vi "openCamera.vi"(0 "error in":errorcluster, 2 "Camera Settings":T2={"Camera"=enum."left_hand_camera", "FPS"=20.0, "Camera Controls"=[{"id"=0, "value"=0}], "Resolution"=enum."(320, 200)"}, 3 "node":string) -> (1 "error out":errorcluster)   [LabVIEW 2012]
doc: "Opens a connection to a Baxter Camera"
uses:
  <userlib>/ROSforLV/ROS/Code/SubVIs/BaxterCamera.ctl
  <userlib>/ROSforLV/ROS/Code/Console/Servers/ServerSubs/TopicDef.ctl
  <userlib>/ROSforLV/ROS/Code/SubVIs/_ROSDirection.ctl
panel:
  out "Reply":string
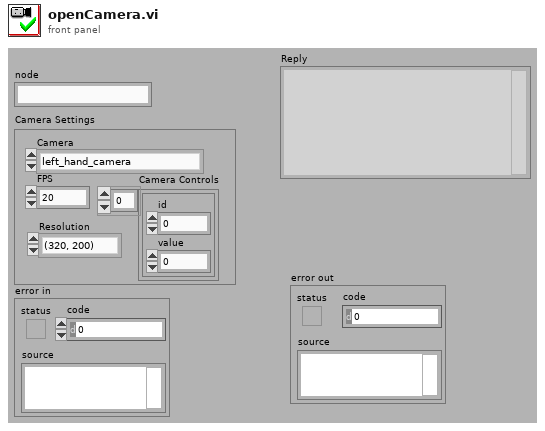
[diagram p1: front panel]
types:
  T1 = typedef "BaxterCamera.ctl" = enum16{"left_hand_camera", "right_hand_camera", "head_camera"}
  T2 = cluster{"Camera":T1, "FPS":sgl, "Camera Controls":cluster{"id":i32, "value":i32}[], "Resolution":enum16{"(1280, 800)", "(960, 600)", "(640, 400)", "(480, 300)", "(384, 240)", "(320, 200)"}}
  T3 = typedef "TopicDef.ctl" = cluster{"Topic":string, "Type":string, "Action":T4, "Update (ms)":u16, "queue size":u16}
  T4 = typedef "_ROSDirection.ctl" = enum16{"Node", "Publisher", "Subscriber", "Service Client"}
  T5 = enum16{"(1280, 800)", "(960, 600)", "(640, 400)", "(480, 300)", "(384, 240)", "(320, 200)"}
  T6 = typedef "_ROSControl.ctl" = cluster{"topic port":u16, "Node":string, "topic":string, "type":string, "node port":u16, "error ":errorcluster, "Direction":T4, "Update (ms)":u16, "queue size":u16}
  T7 = cluster{string, "FPS":sgl, "Camera Controls":cluster{"id":i32, "value":i32}[], "Resolution":enum16{"(1280, 800)", "(960, 600)", "(640, 400)", "(480, 300)", "(384, 240)", "(320, 200)"}}
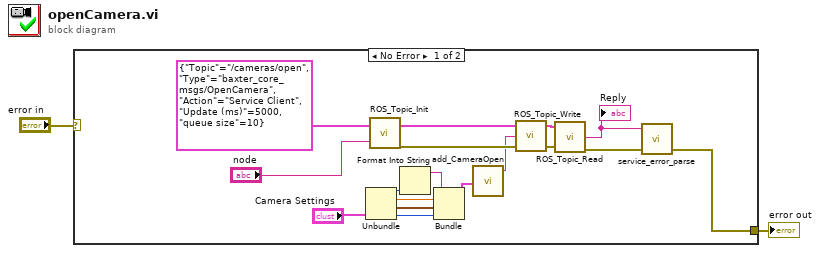
[diagram p0: block diagram]
diagram:
  n1 = case shown="No Error" "error in" {
    selector: "error in" -> [_ w20]
    tunnel: [w3 w20] -> w2
    frame No Error {
      n2 = Unbundle("Camera Settings") -> ("Camera"=w10:T1, "FPS"=w11:sgl, "Camera Controls"=w12:cluster{"id":i32, "value":i32}[], "Resolution"=w13:T5)
      n3 = call <userlib>:"ROS_Topic_Init.vi"("node"="node", "Definitions"=T3 {"Topic"="/cameras/open", "Type"="baxter_core_msgs/OpenCamera", "Action"=enum."Service Client", "Update (ms)"=5000, "queue size"=10}) -> ("error out"=w7:errorcluster, "ROS out"=w18:T6)
      n4 = Format Into String(w10) -> (resulting string=w9:string)  [unwired: 3 in, 1 out]
      n5 = Bundle(w9, "FPS"=w11, "Camera Controls"=w12, "Resolution"=w13) -> (w8:T7)  [unwired: 1 in]
      n6 = call <userlib>:"add_CameraOpen.vi"("Camera Settings"=w8) -> ("msg out"=w5:string)  [unwired: 4 in]
      n7 = call <userlib>:"ROS_Topic_Write.vi"("error in (no error)"=w7, "Msg in"=w5, "ROS in"=w18) -> ("error out"=w6:errorcluster, "ROS out"=w16:T6)  [unwired: 1 in]
      n8 = call <userlib>:"ROS_Topic_Read.vi"("error in (no error)"=w6, "ROS in"=w16) -> ("error out"=w4:errorcluster, "Reply"=w15:string)  [unwired: 1 in, 1 out]
      "Reply" <- w15
      n9 = call <userlib>:"service_error_parse.vi"("error in (no error)"=w4, "Reply"=w15) -> ("error out"=w3:errorcluster)  [unwired: 1 in, 2 out]
    }
    frame Error {
    }
  }
  "error out" <- w2
